vi "Fit Gaussien.vi"(8 "error in (no error)":errorcluster caption="entrée d'erreur (pas d'erreur)", 10 "Signal Autocco":dbl[](array[numeric]), 11 "UI SA en entrée":refnum<class "UI SmarAct.lvclass">) -> (0 "error out":errorcluster caption="sortie d'erreur", 1 "Best Gaussian Fit":dbl[](array[numeric]), 2 "Signal Autocco Norm":dbl[](array[numeric]), 3 "UI SA en sortie":refnum<class "UI SmarAct.lvclass">, 4 "FWHM(Gauss)":dbl, 5 "FWHM(Sech2)":dbl)   [LabVIEW 2024, in "UI SmarAct.lvclass"]
uses:
  UI SmarAct.lvclass
  UI SmarAct.lvclass/UI SmarAct.ctl
  <vilib>/Analysis/NI_AALPro.lvlib
  <vilib>/Analysis/6fits.llb/Curve Fitting Criteria.ctl
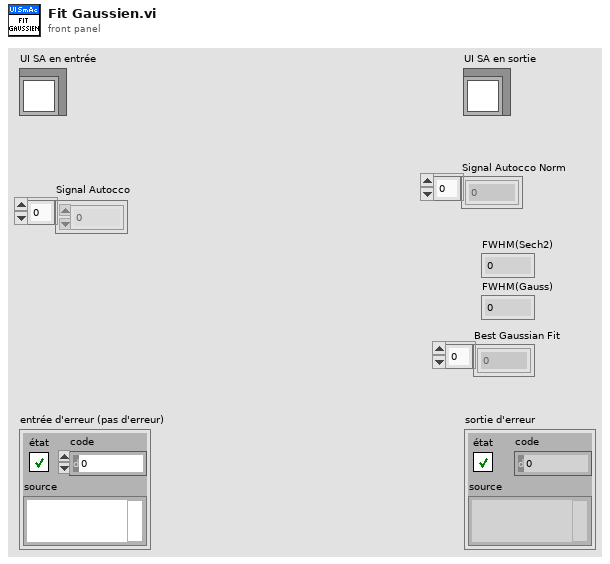
[diagram p1: front panel]
types:
  T1 = typedef "NI_AALPro.lvlib/Curve Fitting Criteria.ctl" = u16
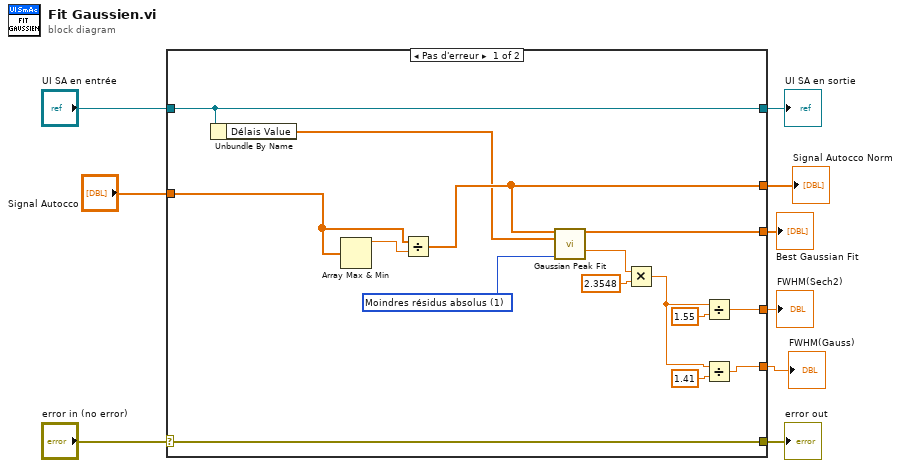
[diagram p0: block diagram]
diagram:
  n1 = case shown="Pas d'erreur" "error in (no error)" {
    selector: "error in (no error)" -> [w24 w27]
    tunnel: [w24 w27] -> w8
    tunnel: [w19 w26] -> w6
    tunnel: "UI SA en entrée" -> [w19 w26]
    tunnel: "Signal Autocco" -> [w22 w25]
    tunnel: [w20 w25] -> w4
    tunnel: [w14 _] -> w3
    tunnel: [w11 _] -> w2
    tunnel: [w10 _] -> w1
    frame No Error {
      w21 = T1 1 items=["Moindres carrés", "Moindres résidus absolus", "Bicarrée"] ("method")
      n2 = Unbundle By Name(w19) -> ("Délais Value"=w18:dbl[])
      n3 = Array Max & Min(array=w22) -> (max value=w23:dbl)  [unwired: 3 out]
      n4 = Divide(x=w22, y=w23) -> (x/y=w20:dbl[])
      n5 = call <vilib>:"Gaussian Peak Fit.vi"("Y"=w20, "X"=w18, "method"=w21) -> ("Best Gaussian Fit"=w10:dbl[], "standard deviation"=w15:dbl)  [unwired: 6 in, 5 out]
      n6 = Multiply(x=w15, y=2.3548) -> (x*y=w12:dbl)
      n7 = Divide(x=w12, y=1.55) -> (x/y=w14:dbl)
      n8 = Divide(x=w12, y=1.41) -> (x/y=w11:dbl)
    }
    frame Error {
    }
  }
  "error out" <- w8
  "UI SA en sortie" <- w6
  "Signal Autocco Norm" <- w4
  "FWHM(Sech2)" <- w3
  "FWHM(Gauss)" <- w2
  "Best Gaussian Fit" <- w1
